vi "Create_Alignment_Event.vi"(4 "Slave data":u8[](array[numeric]), 6 "Master data":u8[](array[numeric]), 8 "Status/Errors in":refnum<vi>, 10 "Process data parameters in":T1={"Stop loop"={"Settings changed?"=FALSE, "Stop?"=refnum}, "Button refs"={"Stop program"=refnum, "Save settings"=refnum, "DAQ mode"=refnum, "Reset settings"=refnum, "Apply settings"=refnum, "Reset MAS"=refnum, "Reset SLV"=refnum, "Local DBase?"=refnum, "Last value DBase"=FALSE, "Database"=refnum, "Calibration"=refnum, "Save settings 2"=refnum}, "Process messages"={"Process message mode"=enum."Error", "Slave data?"=FALSE, "Length get settings message"=0, "Delta time"=0.0, "Data_Filter"={"Filter_Data"=FALSE, "Use_Thresh"=FALSE, "Reduce data?"=FALSE}, "Time_difference_stack"=[], "Starting sec"=0, "Ending sec"=0, "Ending sec 2"=0, "MAS_Page_Thresh"=refnum, "SLV_Page_Thresh"=refnum, "Database"=refnum}, "Settings state"={"MAS locked?"=refnum, "SLV locked?"=refnum}, "Mode"={"Mode"=enum."Dialog", "Expert?"=FALSE, "Dialog?"=FALSE}, "Alignment parameters"=refnum, "Timer parameters"=refnum, "Files"={"Path config file"=path "", "Path def. ini file"=path "", "Path ini file 1"=path "", "Path ini file 2"=path "", "Path RBF file"=path ""}, "Time difference"=refnum, "Alignment"={"GEN_Page_Calibrate"=refnum, "MAS_Page_Gain"=refnum, "MAS_Page_Offset"=refnum, "SLV_Page_Gain"=refnum, "SLV_Page_Offset"=refnum, "MAS_Page_Common"=refnum, "SLV_Page_Common"=refnum}, "Page Statistics"=refnum}) -> (0 "Status/Errors out":refnum<vi>, 2 "Process data parameters out":T1={"Stop loop"={"Settings changed?"=FALSE, "Stop?"=refnum}, "Button refs"={"Stop program"=refnum, "Save settings"=refnum, "DAQ mode"=refnum, "Reset settings"=refnum, "Apply settings"=refnum, "Reset MAS"=refnum, "Reset SLV"=refnum, "Local DBase?"=refnum, "Last value DBase"=FALSE, "Database"=refnum, "Calibration"=refnum, "Save settings 2"=refnum}, "Process messages"={"Process message mode"=enum."Error", "Slave data?"=FALSE, "Length get settings message"=0, "Delta time"=0.0, "Data_Filter"={"Filter_Data"=FALSE, "Use_Thresh"=FALSE, "Reduce data?"=FALSE}, "Time_difference_stack"=[], "Starting sec"=0, "Ending sec"=0, "Ending sec 2"=0, "MAS_Page_Thresh"=refnum, "SLV_Page_Thresh"=refnum, "Database"=refnum}, "Settings state"={"MAS locked?"=refnum, "SLV locked?"=refnum}, "Mode"={"Mode"=enum."Dialog", "Expert?"=FALSE, "Dialog?"=FALSE}, "Alignment parameters"=refnum, "Timer parameters"=refnum, "Files"={"Path config file"=path "", "Path def. ini file"=path "", "Path ini file 1"=path "", "Path ini file 2"=path "", "Path RBF file"=path ""}, "Time difference"=refnum, "Alignment"={"GEN_Page_Calibrate"=refnum, "MAS_Page_Gain"=refnum, "MAS_Page_Offset"=refnum, "SLV_Page_Gain"=refnum, "SLV_Page_Offset"=refnum, "MAS_Page_Common"=refnum, "SLV_Page_Common"=refnum}, "Page Statistics"=refnum})   [LabVIEW 2013]
uses:
  Controls/Process_Data_Parameters.ctl
  Controls/Stop_Loop.ctl
  Controls/Button_Refs.ctl
  Controls/Process_Messages.ctl
  Controls/Process_Message_Mode.ctl
  Controls/Settings_State.ctl
  Controls/Mode.ctl
  Controls/Files.ctl
  Controls/Page_Calibration.ctl
  Controls/Get_Set_Calibration_Options.ctl
  Controls/Master.ctl
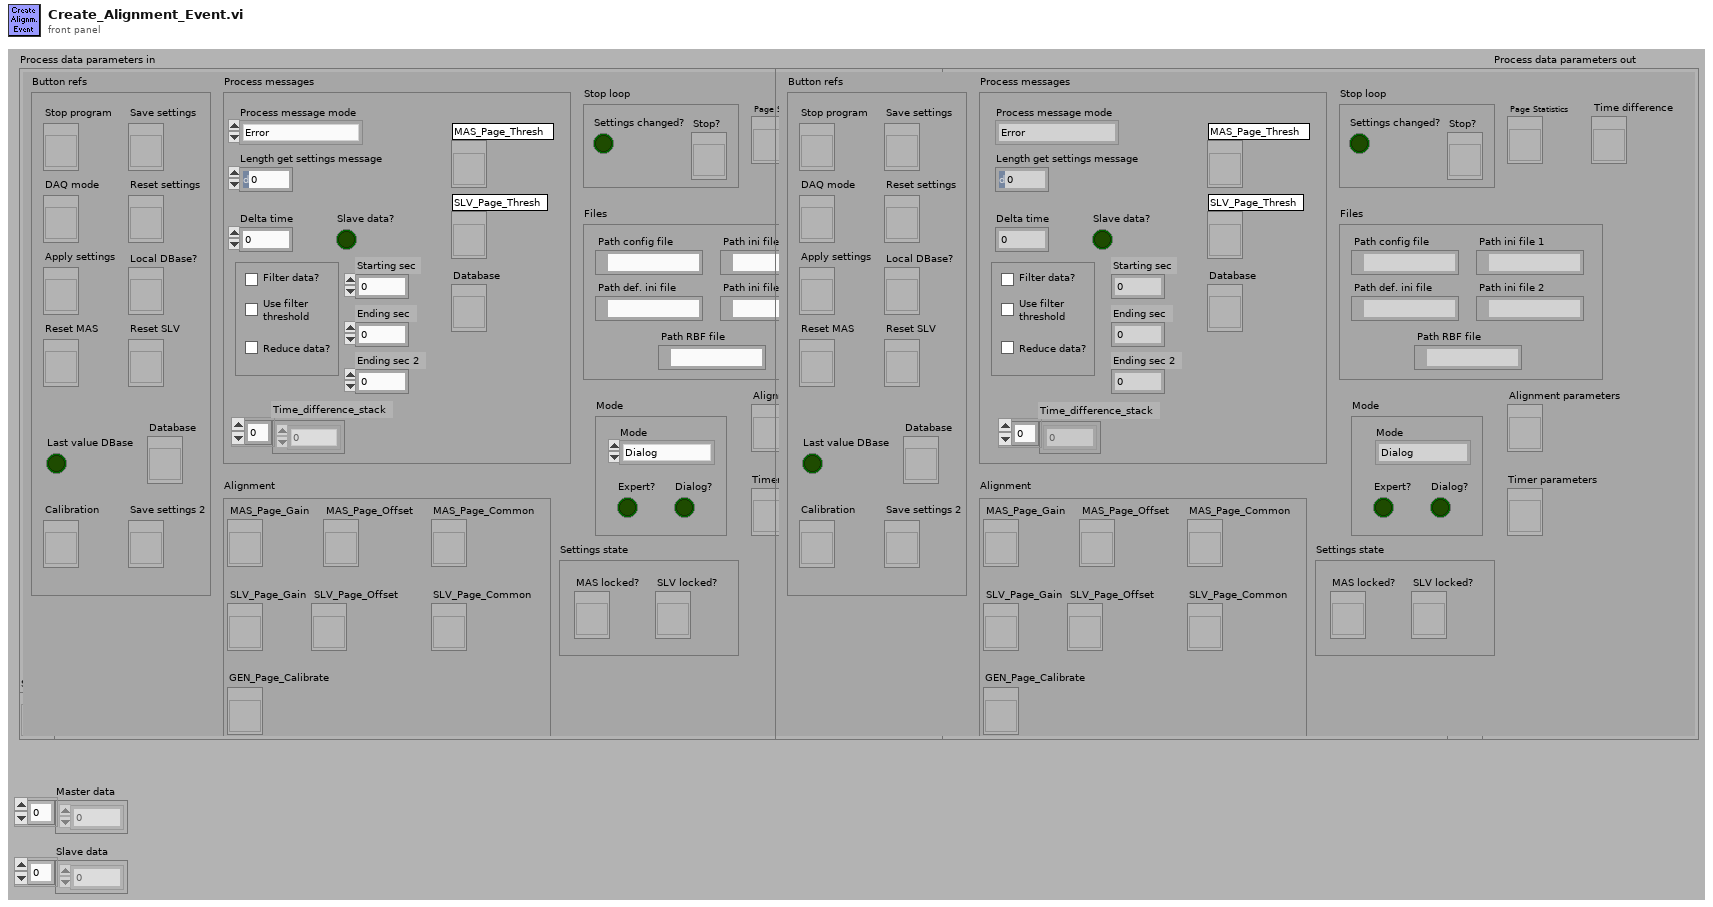
[diagram p1: front panel]
types:
  T1 = typedef "Process_Data_Parameters.ctl" = cluster{"Stop loop":T2, "Button refs":T3, "Process messages":T4, "Settings state":T6, "Mode":T7, "Alignment parameters":refnum<vi>, "Timer parameters":refnum<vi>, "Files":T8, "Time difference":refnum<vi>, "Alignment":T9, "Page Statistics":refnum<vi>}
  T2 = typedef "Stop_Loop.ctl" = cluster{"Settings changed?":bool, "Stop?":refnum<vi>}
  T3 = typedef "Button_Refs.ctl" = cluster{"Stop program":refnum<vi>, "Save settings":refnum<vi>, "DAQ mode":refnum<vi>, "Reset settings":refnum<vi>, "Apply settings":refnum<vi>, "Reset MAS":refnum<vi>, "Reset SLV":refnum<vi>, "Local DBase?":refnum<vi>, "Last value DBase":bool, "Database":refnum<vi>, "Calibration":refnum<vi>, "Save settings 2":refnum<vi>}
  T4 = typedef "Process_Messages.ctl" = cluster{"Process message mode":T5, "Slave data?":bool, "Length get settings message":i32, "Delta time":dbl, "Data_Filter":cluster{"Filter_Data":bool, "Use_Thresh":bool, "Reduce data?":bool}, "Time_difference_stack":u64[], "Starting sec":u64, "Ending sec":u64, "Ending sec 2":u64, "MAS_Page_Thresh":refnum<vi>, "SLV_Page_Thresh":refnum<vi>, "Database":refnum<vi>}
  T5 = typedef "Process_Message_Mode.ctl" = enum16{"Error", "Measurement data", "Comparator data", "One Second"}
  T6 = typedef "Settings_State.ctl" = cluster{"MAS locked?":refnum<vi>, "SLV locked?":refnum<vi>}
  T7 = typedef "Mode.ctl" = cluster{"Mode":enum8{"Stop", "Dialog", "Hisparc II", "Hisparc II DAQ", "Alignment"}, "Expert?":bool, "Dialog?":bool}
  T8 = typedef "Files.ctl" = cluster{"Path config file":path, "Path def. ini file":path, "Path ini file 1":path, "Path ini file 2":path, "Path RBF file":path}
  T9 = typedef "Page_Calibration.ctl" = cluster{"GEN_Page_Calibrate":refnum<vi>, "MAS_Page_Gain":refnum<vi>, "MAS_Page_Offset":refnum<vi>, "SLV_Page_Gain":refnum<vi>, "SLV_Page_Offset":refnum<vi>, "MAS_Page_Common":refnum<vi>, "SLV_Page_Common":refnum<vi>}
  T10 = typedef "Get_Set_Calibration_Options.ctl" = enum16{"Get", "Set", "Set MAS", "Set SLV"}
  T11 = typedef "Master.ctl" = enum16{"Master", "Slave", "General"}
  T12 = typedef "Calibration_Parameters.ctl" = cluster{"New settings MAS?":bool, "New settings SLV?":bool, "Alignment step MAS":i32, "Alignment step SLV":i32, "MAS Ch. 1":cluster{"Offset adjust pos.":u8, "Offset adjust neg.":u8, "Gain adjust pos.":u8, "Gain adjust neg.":u8, "Count pos.":dbl, "Count neg.":dbl}, "MAS Ch. 2":cluster{"Offset adjust pos.":u8, "Offset adjust neg.":u8, "Gain adjust pos.":u8, "Gain adjust neg.":u8, "Count pos.":dbl, "Count neg.":dbl}, "SLV Ch. 1":cluster{"Offset adjust pos.":u8, "Offset adjust neg.":u8, "Gain adjust pos.":u8, "Gain adjust neg.":u8, "Count pos.":dbl, "Count neg.":dbl}, "SLV Ch. 2":cluster{"Offset adjust pos.":u8, "Offset adjust neg.":u8, "Gain adjust pos.":u8, "Gain adjust neg.":u8, "Count pos.":dbl, "Count neg.":dbl}, "Comm. offset MAS":u8, "Full scale MAS":u8, "Comm. offset SLV":u8, "Full scale SLV":u8, "Trigger condition":u8, "Pre coinc. time":u16, "Coinc. time":u16, "Post coinc. time":u16, "Hardware":enum8{"None", "HiSPARC I", "HiSPARC II", "HiSPARC III", "Unknown"}}
  T13 = cluster{"Calibration":bool, "Traces":dbl[][], "Calibration_step_MAS":i32, "Calibration_step_SLV":i32, "Voltage_adjust_MAS":u8, "Voltage_adjust_SLV":u8}
  T14 = cluster{"Ch1_Gain_Pos":u8, "Ch1_Gain_Neg":u8, "Ch2_Gain_Pos":u8, "Ch2_Gain_Neg":u8}
  T15 = cluster{"Ch1_Offset_Pos":u8, "Ch1_Offset_Neg":u8, "Ch2_Offset_Pos":u8, "Ch2_Offset_Neg":u8}
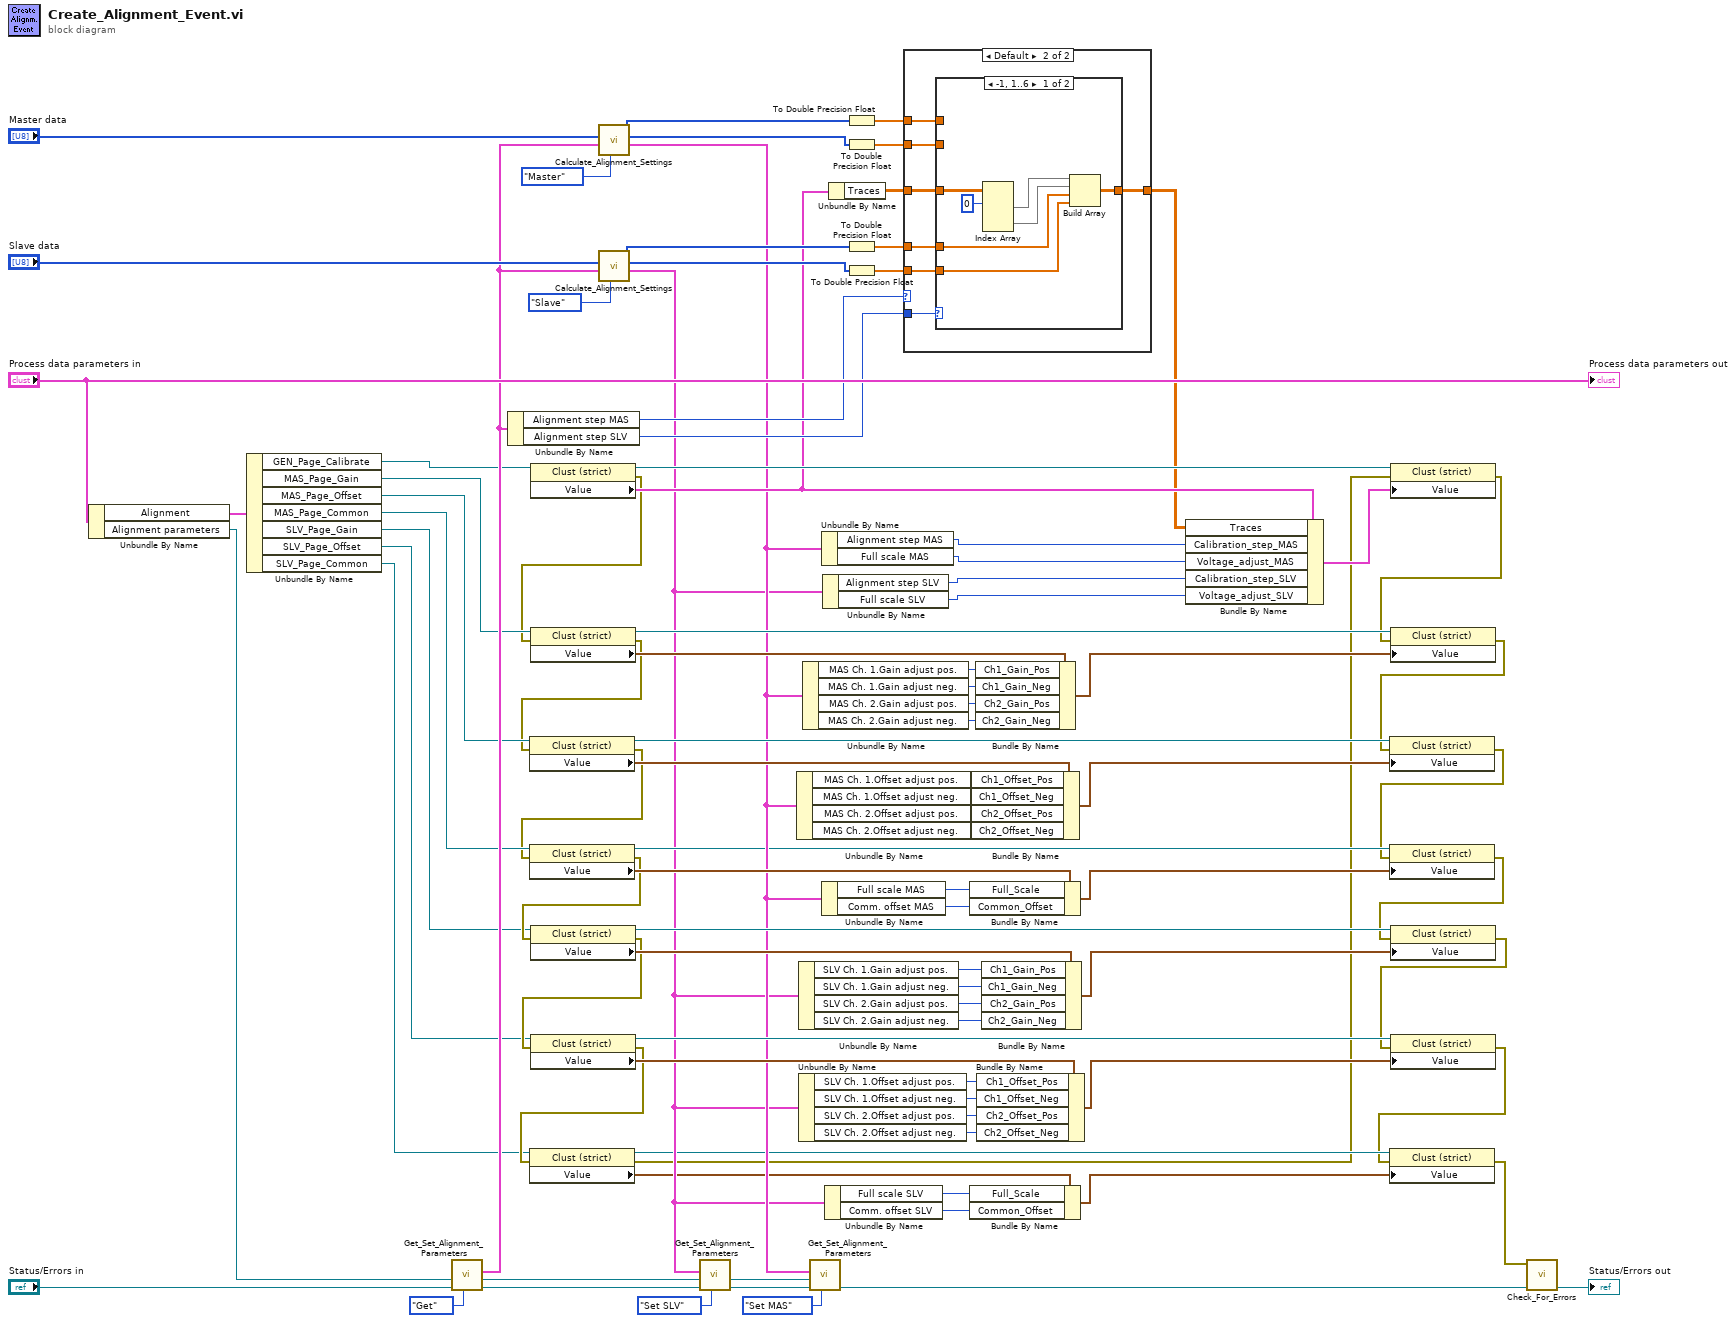
[diagram p0: block diagram]
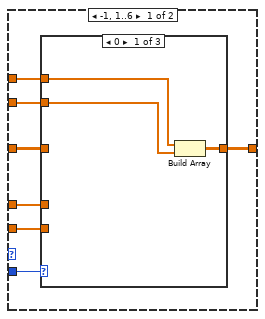
[diagram p2: hidden frame]
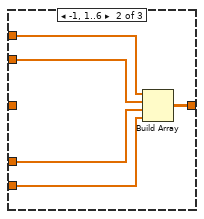
[diagram p3: hidden frame]
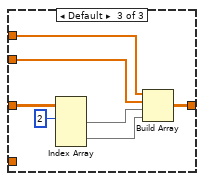
[diagram p4: hidden frame]
diagram:
  n1 = Unbundle By Name("Process data parameters in") -> ("Alignment"=w61:T9, "Alignment parameters"=w98:refnum<vi>)
  n2 = Unbundle By Name(w61) -> ("GEN_Page_Calibrate"=w66:refnum<vi>, "MAS_Page_Gain"=w60:refnum<vi>, "MAS_Page_Offset"=w59:refnum<vi>, "MAS_Page_Common"=w20:refnum<vi>, "SLV_Page_Gain"=w3:refnum<vi>, "SLV_Page_Offset"=w2:refnum<vi>, "SLV_Page_Common"=w1:refnum<vi>)
  n3 = call "Get_Set_Alignment_Parameters.vi"("Get/Set"=Get_Set_Calibration_Options."Get", "Status/Errors in"="Status/Errors in", "Alignment parameters in"=w98) -> ("Status/Errors out"=w62:refnum<vi>, "Alignment parameters out"=w95:refnum<vi>, "Value out"=w82:T12)  [unwired: 2 in, 4 out]
  n4 = Unbundle By Name(w82) -> ("Alignment step MAS"=w78:i32, "Alignment step SLV"=w77:i32)
  n5 = property class="Clust (strict)"(reference=w66) -> (reference out=w86:refnum<vi>, error out=w27:errorcluster, "Value"=w72:T13)  [unwired: 1 in]
  n6 = property class="Clust (strict)"(reference=w60, error in=w27) -> (reference out=w38:refnum<vi>, error out=w26:errorcluster, "Value"=w43:T14)
  n7 = property class="Clust (strict)"(reference=w59, error in=w26) -> (reference out=w37:refnum<vi>, error out=w19:errorcluster, "Value"=w48:T15)
  n8 = property class="Clust (strict)"(reference=w20, error in=w19) -> (reference out=w16:refnum<vi>, error out=w18:errorcluster, "Value"=w24:cluster{"Full_Scale":u8, "Common_Offset":u8})
  n9 = property class="Clust (strict)"(reference=w3, error in=w18) -> (reference out=w36:refnum<vi>, error out=w25:errorcluster, "Value"=w58:T14)
  n10 = property class="Clust (strict)"(reference=w2, error in=w25) -> (reference out=w35:refnum<vi>, error out=w5:errorcluster, "Value"=w53:T15)
  n11 = property class="Clust (strict)"(reference=w1, error in=w5) -> (reference out=w9:refnum<vi>, error out=w4:errorcluster, "Value"=w10:cluster{"Full_Scale":u8, "Common_Offset":u8})
  n12 = call "Calculate_Alignment_Settings.vi"("Master?"=Master."Master", "Alignment parameters in"=w82, "Data"="Master data") -> ("Alignment parameters out"=w17:T12, "Data ch. 2"=w79:u16[], "Data ch.1"=w70:u16[])  [unwired: 2 in, 4 out]
  n13 = call "Calculate_Alignment_Settings.vi"("Master?"=Master."Slave", "Alignment parameters in"=w82, "Data"="Slave data") -> ("Alignment parameters out"=w11:T12, "Data ch. 2"=w80:u16[], "Data ch.1"=w81:u16[])  [unwired: 2 in, 4 out]
  n14 = call "Get_Set_Alignment_Parameters.vi"("Get/Set"=Get_Set_Calibration_Options."Set SLV", "Status/Errors in"=w62, "Alignment parameters in"=w95, "Value in"=w11) -> ("Status/Errors out"=w92:refnum<vi>, "Alignment parameters out"=w93:refnum<vi>)  [unwired: 1 in, 5 out]
  n15 = Unbundle By Name(w17) -> ("MAS Ch. 1.Offset adjust pos."=w47:u8, "MAS Ch. 1.Offset adjust neg."=w46:u8, "MAS Ch. 2.Offset adjust pos."=w45:u8, "MAS Ch. 2.Offset adjust neg."=w44:u8)
  n16 = Unbundle By Name(w11) -> ("SLV Ch. 1.Gain adjust pos."=w57:u8, "SLV Ch. 1.Gain adjust neg."=w56:u8, "SLV Ch. 2.Gain adjust pos."=w55:u8, "SLV Ch. 2.Gain adjust neg."=w54:u8)
  n17 = Unbundle By Name(w11) -> ("SLV Ch. 1.Offset adjust pos."=w52:u8, "SLV Ch. 1.Offset adjust neg."=w51:u8, "SLV Ch. 2.Offset adjust pos."=w50:u8, "SLV Ch. 2.Offset adjust neg."=w49:u8)
  n18 = Unbundle By Name(w17) -> ("MAS Ch. 1.Gain adjust pos."=w42:u8, "MAS Ch. 1.Gain adjust neg."=w41:u8, "MAS Ch. 2.Gain adjust pos."=w40:u8, "MAS Ch. 2.Gain adjust neg."=w39:u8)
  n19 = call "Get_Set_Alignment_Parameters.vi"("Get/Set"=Get_Set_Calibration_Options."Set MAS", "Status/Errors in"=w92, "Alignment parameters in"=w93, "Value in"=w17) -> ("Status/Errors out"=w85:refnum<vi>)  [unwired: 1 in, 6 out]
  n20 = Unbundle By Name(w17) -> ("Alignment step MAS"=w83:i32, "Full scale MAS"=w65:u8)
  n21 = Unbundle By Name(w17) -> ("Full scale MAS"=w23:u8, "Comm. offset MAS"=w22:u8)
  n22 = Unbundle By Name(w11) -> ("Alignment step SLV"=w64:i32, "Full scale SLV"=w63:u8)
  n23 = Unbundle By Name(w11) -> ("Full scale SLV"=w13:u8, "Comm. offset SLV"=w12:u8)
  n24 = Unbundle By Name(w72) -> ("Traces"=w68:dbl[][])
  n25 = To Double Precision Float(number=w70) -> (double precision float=w73:dbl[])
  n26 = To Double Precision Float(number=w79) -> (double precision float=w74:dbl[])
  n27 = To Double Precision Float(number=w81) -> (double precision float=w75:dbl[])
  n28 = To Double Precision Float(number=w80) -> (double precision float=w76:dbl[])
  n29 = case shown="Default" w78 {
    tunnel: w77 -> [w105 w127]
    tunnel: w76 -> [w104 w126]
    tunnel: w75 -> [w103 w125]
    tunnel: w74 -> [w102 w124]
    tunnel: w73 -> [w101 w123]
    tunnel: [w100 w122] -> w67
    tunnel: w68 -> [w99 w121]
    frame -1, 1..6 {
      n30 = case shown="0" w105 {
        tunnel: w104 -> [_ w110 _]
        tunnel: w103 -> [_ w111 _]
        tunnel: w102 -> [w107 w112 w119]
        tunnel: w101 -> [w108 w113 w120]
        tunnel: [w106 w109 w118] -> w100
        tunnel: w99 -> [_ _ w117]
        frame 0 {
          n31 = Build Array(w108, w107) -> (w106:dbl[][])
        }
        frame -1, 1..6 {
          n32 = Build Array(w113, w112, w111, w110) -> (w109:dbl[][])
        }
        frame Default {
          n33 = Index Array(array=w117, index (row) #1=2 ("index (row)")) -> (element #1=w115:dbl[], element #2=w114:dbl[])  [unwired: 3 in]
          n34 = Build Array(w120, w119, w115, w114) -> (w118:dbl[][])
        }
      }
    }
    frame Default {
      n35 = case shown="-1, 1..6" w127 {
        tunnel: w126 -> [w128 _]
        tunnel: w125 -> [w129 _]
        tunnel: w124 -> [_ _]
        tunnel: w123 -> [_ _]
        tunnel: [w134 w135] -> w122
        tunnel: w121 -> [w133 w135]
        frame -1, 1..6 {
          n36 = Index Array(array=w133, index (row) #1=0 ("index (row)")) -> (element #1=w131:dbl[], element #2=w130:dbl[])  [unwired: 3 in]
          n37 = Build Array(w131, w130, w129, w128) -> (w134:dbl[][])
        }
        frame Default {
        }
      }
    }
  }
  n38 = Bundle By Name(cluster=w24, "Full_Scale"=w23, "Common_Offset"=w22) -> (w21:cluster{"Full_Scale":u8, "Common_Offset":u8})
  n39 = Bundle By Name(cluster=w10, "Full_Scale"=w13, "Common_Offset"=w12) -> (w8:cluster{"Full_Scale":u8, "Common_Offset":u8})
  n40 = Bundle By Name(cluster=w48, "Ch1_Offset_Pos"=w47, "Ch1_Offset_Neg"=w46, "Ch2_Offset_Pos"=w45, "Ch2_Offset_Neg"=w44) -> (w33:T15)
  n41 = Bundle By Name(cluster=w43, "Ch1_Gain_Pos"=w42, "Ch1_Gain_Neg"=w41, "Ch2_Gain_Pos"=w40, "Ch2_Gain_Neg"=w39) -> (w34:T14)
  n42 = Bundle By Name(cluster=w53, "Ch1_Offset_Pos"=w52, "Ch1_Offset_Neg"=w51, "Ch2_Offset_Pos"=w50, "Ch2_Offset_Neg"=w49) -> (w31:T15)
  n43 = Bundle By Name(cluster=w58, "Ch1_Gain_Pos"=w57, "Ch1_Gain_Neg"=w56, "Ch2_Gain_Pos"=w55, "Ch2_Gain_Neg"=w54) -> (w32:T14)
  n44 = Bundle By Name(cluster=w72, "Traces"=w67, "Calibration_step_MAS"=w83, "Voltage_adjust_MAS"=w65, "Calibration_step_SLV"=w64, "Voltage_adjust_SLV"=w63) -> (w87:T13)
  n45 = property class="Clust (strict)"(reference=w86, error in=w4, "Value"=w87) -> (error out=w30:errorcluster)  [unwired: 1 out]
  n46 = property class="Clust (strict)"(reference=w38, error in=w30, "Value"=w34) -> (error out=w29:errorcluster)  [unwired: 1 out]
  n47 = property class="Clust (strict)"(reference=w37, error in=w29, "Value"=w33) -> (error out=w15:errorcluster)  [unwired: 1 out]
  n48 = property class="Clust (strict)"(reference=w16, error in=w15, "Value"=w21) -> (error out=w14:errorcluster)  [unwired: 1 out]
  n49 = property class="Clust (strict)"(reference=w36, error in=w14, "Value"=w32) -> (error out=w28:errorcluster)  [unwired: 1 out]
  n50 = property class="Clust (strict)"(reference=w35, error in=w28, "Value"=w31) -> (error out=w7:errorcluster)  [unwired: 1 out]
  n51 = property class="Clust (strict)"(reference=w9, error in=w7, "Value"=w8) -> (error out=w6:errorcluster)  [unwired: 1 out]
  n52 = call "Check_For_Errors.vi"("Status/Errors in"=w85, "error in"=w6) -> ("Status/Errors out"=→"Status/Errors out":refnum<vi>)  [unwired: 9 out]
  "Process data parameters out" <- "Process data parameters in"
